vi "Init.vi"(8 "error in":errorcluster) -> (0 "error out":errorcluster)   [LabVIEW 2015, in "Generic Module Library.lvlib" / "Template G_Module.lvlib"]
uses:
  Template G_Module.lvlib
  Private Controls/Module Message Cluster Components/Message Data Cluster.ctl
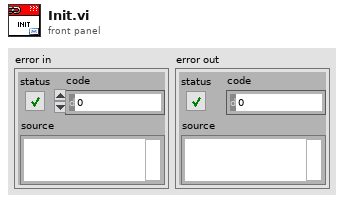
[diagram p1: front panel]
types:
  T1 = typedef "Generic Module Library.lvlib/Template G_Module.lvlib/Message Data Cluster.ctl" = cluster{"Module Action":string, "Message Data":variant}
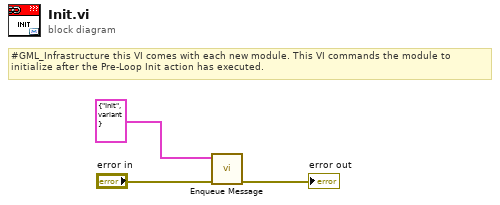
[diagram p0: block diagram]
diagram:
  # "#GML_Infrastructure this VI comes with each new module. This VI commands the module to initialize after the Pre-Loop Init action has executed."
  n1 = call "Enqueue Message.vi"("error in"="error in", "Message Data"=T1 {"Module Action"="Init", "Message Data"=variant}) -> ("error out"=→"error out":errorcluster)  [unwired: 9 in]
